vi "SeqMap_Get.vi"(8 "error in (no error)":errorcluster) -> (0 "error out":errorcluster, 3 "SeqMap":T1)   [LabVIEW 2016, in "SeqProcessor.lvlib"]
uses:
  SeqProcessor.lvlib
  <vilib>/addons/PointValueMap/controls/PointMap.ctl
  <vilib>/addons/PointValueMap/PointValueMap.lvlib
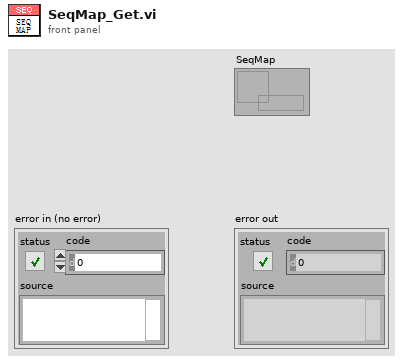
[diagram p1: front panel]
types:
  T1 = typedef "PointValueMap.lvlib/PointMap.ctl" = refnum<data-value>
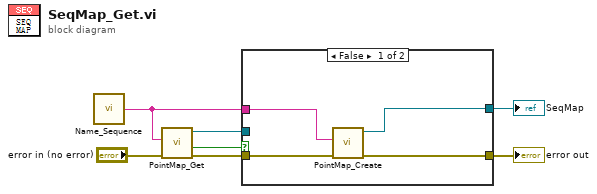
[diagram p0: block diagram]
diagram:
  n1 = call "Name_Sequence.vi"() -> ("SequenceName"=w1:string)  [unwired: 5 in]
  n2 = call <vilib>:"PointMap_Get.vi"("error in (no error)"="error in (no error)", "Name"=w1) -> ("error out"=w5:errorcluster, "Found?"=w6:bool, "Map Out"=w2:T1)  [unwired: 7 in]
  n3 = case shown="False" w6 {
    tunnel: w5 -> [w11 w12]
    tunnel: [w10 w12] -> w4
    tunnel: [w9 w13] -> w3
    tunnel: w2 -> [_ w13]
    tunnel: w1 -> [w8 _]
    frame False {
      n4 = call <vilib>:"PointMap_Create.vi"("error in (no error)"=w11, "Name"=w8) -> ("error out"=w10:errorcluster, "Map Out"=w9:T1)  [unwired: 8 in]
    }
    frame True {
    }
  }
  "error out" <- w4
  "SeqMap" <- w3
